vi "长轴.vi"(8 "y2":dbl, 9 "x2":dbl, 10 "y1":dbl, 11 "x1":dbl) -> (1 "长轴长度":dbl, 2 "第二点x值，y=479":dbl, 3 "第一点x值，y=0":dbl)   [LabVIEW 2015]
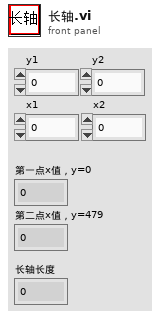
[diagram p1: front panel]
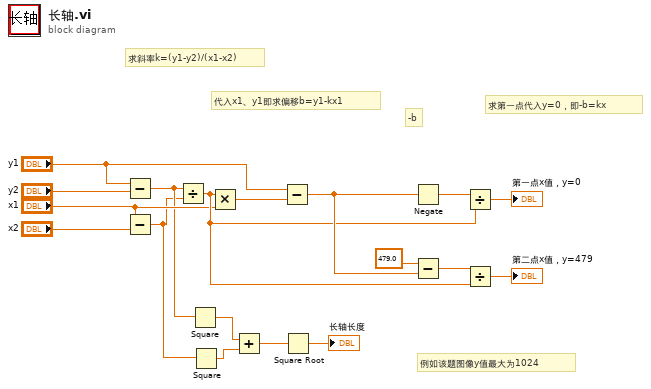
[diagram p0: block diagram]
diagram:
  # "例如该题图像y值最大为1024"
  # "-b"
  # "求第一点代入y=0，即-b=kx"
  # "代入x1、y1即求偏移b=y1-kx1"
  # "求斜率k=(y1-y2)/(x1-x2)"
  n1 = Subtract(x="y1", y="y2") -> (x-y=w6:dbl)
  n2 = Subtract(x="x1", y="x2") -> (x-y=w3:dbl)
  n3 = Divide(x=w6, y=w3) -> (x/y=w11:dbl)
  n4 = Square(x=w6) -> (x^2=w5:dbl)
  n5 = Square(x=w3) -> (x^2=w4:dbl)
  n6 = Multiply(x=w11, y="x1") -> (x*y=w12:dbl)
  n7 = Add(x=w5, y=w4) -> (x+y=w2:dbl)
  n8 = Subtract(x="y1", y=w12) -> (x-y=w16:dbl)
  n9 = Square Root(x=w2) -> (sqrt(x)=→"长轴长度":dbl)
  n10 = Negate(x=w16) -> (-x=w18:dbl)
  n11 = Subtract(x=479.0, y=w16) -> (x-y=w15:dbl)
  n12 = Divide(x=w18, y=w11) -> (x/y=→"第一点x值，y=0":dbl)
  n13 = Divide(x=w15, y=w11) -> (x/y=→"第二点x值，y=479":dbl)
